vi "Write Tag Value_ByRef.vi"(5 "IgnoreIfEqual (F)":bool, 7 "Timestamp (now)":timestamp, 8 "error in (no error)":errorcluster, 9 "Value":variant, 10 "Tag Ref in":refnum<data-value>) -> (0 "error out":errorcluster, 2 "Tag Ref out":refnum<data-value>)   [LabVIEW 2020, in "Tag Engine.lvlib" / "Tag Core.lvclass"]
doc: "_SubVI_"
uses:
  Tag Core.lvclass
  Tag/Tag.lvclass
  Tag/Tag.lvclass/Tag.ctl
  Tag Core.lvclass/Tag Core.ctl
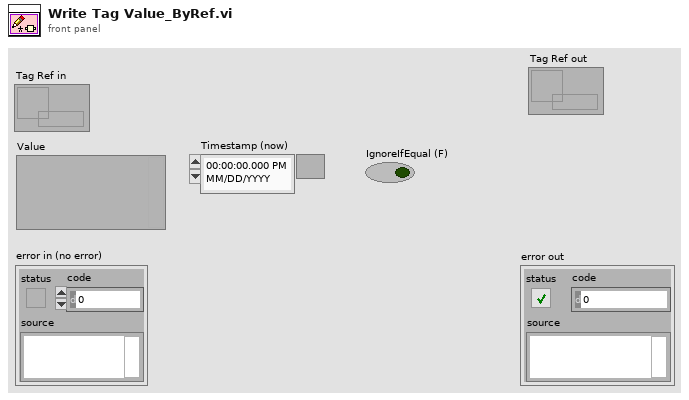
[diagram p1: front panel]
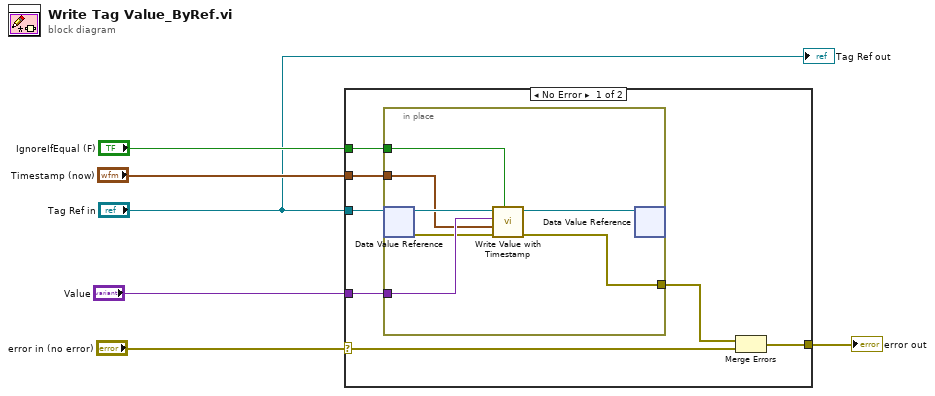
[diagram p0: block diagram]
diagram:
  n1 = case shown="No Error" "error in (no error)" {
    selector: "error in (no error)" -> [w12 w21]
    tunnel: "Tag Ref in" -> [w13 _]
    tunnel: [w11 w21] -> w6
    tunnel: "Value" -> [w10 _]
    tunnel: "Timestamp (now)" -> [w8 _]
    tunnel: "IgnoreIfEqual (F)" -> [w7 _]
    frame No Error {
      n2 = in-place {
        in-place-border: w10 -> [w20]
        in-place-border: [w16] -> w9
        in-place-border: w8 -> [w15]
        in-place-border: w7 -> [w14]
        n3 = in-place-dvr #1(w13) -> (w19:refnum<class "Tag.lvclass">, w17:errorcluster)
        n4 = call "Write Value with Timestamp.vi"("IgnoreIfEqual (F)"=w14, "error in (no error)"=w17, "Timestamp (now)"=w15, "Value"=w20, "Tag in"=w19) -> ("error out"=w16:errorcluster, "Tag out"=w18:refnum<class "Tag.lvclass">)  [unwired: 5 in]
        n5 = in-place-dvr #1(w18) -> ()  [unwired: 2 out]
      }
      n6 = Merge Errors(w9, w12) -> (w11:errorcluster)
    }
    frame Error {
    }
  }
  "error out" <- w6
  "Tag Ref out" <- "Tag Ref in"
